vi "rx Buffer Push LV.vi"(10 "data":u8, 11 "instance":i32) -> (3 "function return":u32)   [LabVIEW 2022 SP3, in "SADI_FW3.lvlib"]
doc: "SADI_API_Wrapper ringBufInfo_t rxBufferPush_LV(int instance, uint8_t data);"
uses:
  SADI_FW3.lvlib
  SADI_FW3.dll
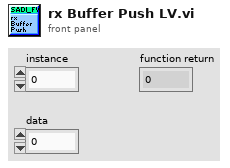
[diagram p1: front panel]
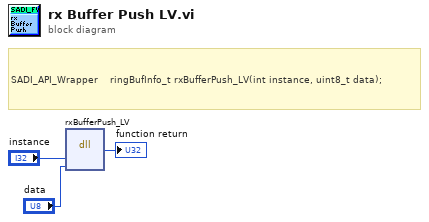
[diagram p0: block diagram]
diagram:
  # "SADI_API_Wrapper    ringBufInfo_t rxBufferPush_LV(int instance, uint8_t data);"
  n1 = dll-call lib="C:/Users/scer/OneDrive - University of Florida/eml4314c/eml4314Sp24/Resources/release_1_11_24/EML4314c_Sp24_framework_0/LVLib/SADI_FW3.*" fn="rxBufferPush_LV"("instance"="instance", "data"="data") -> (→"function return":u32)  [unwired: 5 in, 2 out]
